vi "Read Timeout.vi"(8 "error in":errorcluster, 11 "Popup in":refnum<class "Popup.lvclass">) -> (0 "error out":errorcluster, 2 "Timeout?":bool, 3 "Popup out":refnum<class "Popup.lvclass">)   [LabVIEW 2021, in "Pop-Up.lvlib" / "Popup.lvclass"]
doc: "This Data Member Access VI will read the timeout Boolean from the object.\n\nOutputs\n-Timeout [Boolean] - the timeout result\n\n<b>Code Developed By:</b>\nDaniel Coons\nTechnology Service Corporation\n1983 S Liberty Drive\nBloomington, IN 47403\nPhone: 812 558-7100\ndaniel.coons@tsc.com\nwww.tsc.com/atcs"
uses:
  Popup.lvclass
  Popup.lvclass/Popup.ctl
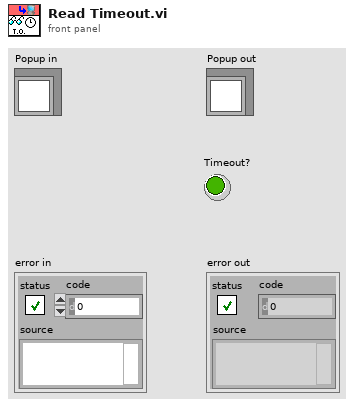
[diagram p1: front panel]
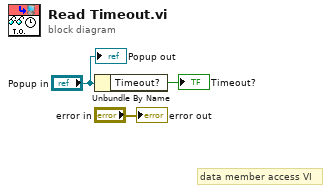
[diagram p0: block diagram]
diagram:
  # "data member access VI"
  n1 = Unbundle By Name("Popup in") -> ("Timeout?"=→"Timeout?":bool)
  "error out" <- "error in"
  "Popup out" <- "Popup in"
